vi "MP-285 Close.vi"(2 "error in (no error)":errorcluster, 3 "VISA resource name":refnum<visa-resource-name>) -> (0 "Output: Error cluster":errorcluster)   [LabVIEW 2010]
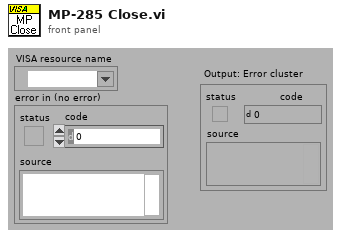
[diagram p1: front panel]
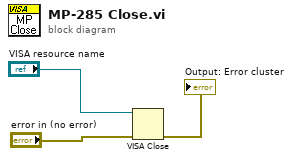
[diagram p0: block diagram]
diagram:
  n1 = VISA Close(VISA resource name="VISA resource name", error in (no error)="error in (no error)") -> (error out=→"Output: Error cluster":errorcluster)
